vi "uActor_ReceiveNestedStopped.vi"(8 "error in (no error)":errorcluster, 10 "uData in":refnum<class "uData.lvclass">, 11 "uActor in":refnum<class "uActor.lvclass">) -> (0 "error out":errorcluster, 3 "uActor out":refnum<class "uActor.lvclass">)   [LabVIEW 2023, in "uLib.lvlib" / "uActor.lvclass"]
uses:
  uActor.lvclass
  uData/uData/uData.lvclass
  uData/uData/uData.lvclass/uData.ctl
  uActor.lvclass/uActor.ctl
  uData/uData/Condition Tag Name.vi
  uData/uData/Blank Key Reserved String.vi
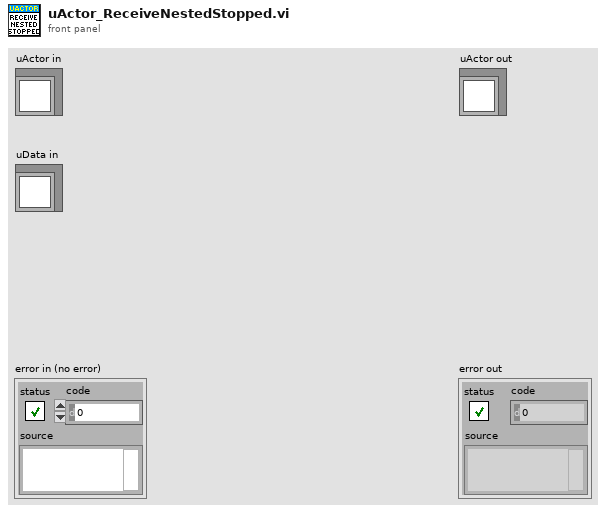
[diagram p1: front panel]
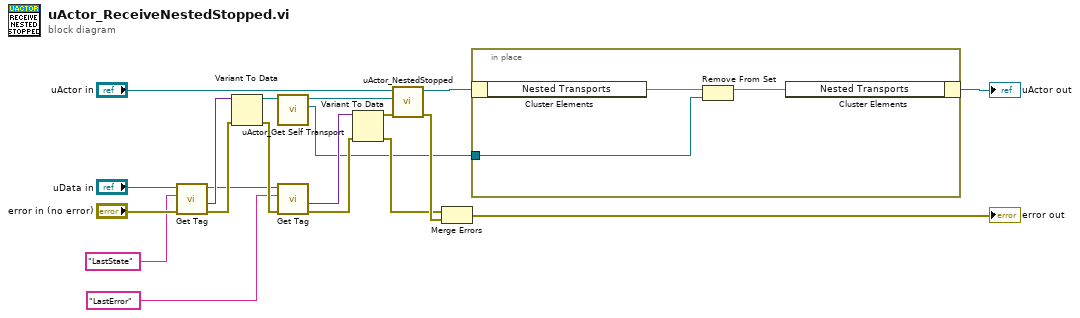
[diagram p0: block diagram]
diagram:
  n1 = call "Get Tag.vi"("error in (no error)"="error in (no error)", "tag (case insensitive)"="LastState" ("uMsg Tag"), "uData in"="uData in") -> ("error out"=w15:errorcluster, "value"=w18:variant, "uData out"=w13:refnum<class "uData.lvclass">)  [unwired: 5 in, 1 out]
  n2 = Variant To Data(error in=w15, Variant=w18) -> (data=w5:refnum<class "uActor.lvclass">, error out=w14:errorcluster)  [unwired: 1 in]
  n3 = call "uActor_Get Self Transport.vi"("uActor in"=w5) -> ("Actor Transport"=w3:refnum<class "uTransport_uActor.lvclass">, "uActor out"=w4:refnum<class "uActor.lvclass">)  [unwired: 9 in]
  n4 = call "Get Tag.vi"("error in (no error)"=w14, "tag (case insensitive)"="LastError" ("uMsg Tag"), "uData in"=w13) -> ("error out"=w12:errorcluster, "value"=w16:variant)  [unwired: 5 in, 2 out]
  n5 = Variant To Data(error in=w12, Variant=w16) -> (data=w17:errorcluster, error out=w11:errorcluster)  [unwired: 1 in]
  n6 = call-dynamic "uActor_NestedStopped.vi"("NestedActor - Last Error"=w17, "NestedActor - Last State"=w4, "uActor in"="uActor in") -> ("error out"=w19:errorcluster, "uActor out"=w7:refnum<class "uActor.lvclass">)  [unwired: 7 in]
  n7 = Merge Errors(w11, w19) -> (→"error out":errorcluster)
  n8 = in-place {
    in-place-border: w3 -> [w21]
    n9 = in-place-cluster #1(w7) -> ("Nested Transports"=w23:set{refnum<class "uTransport_uActor.lvclass">})
    n10 = Remove From Set(10:w21, 11:w23) -> (3:w22:set{refnum<class "uTransport_uActor.lvclass">})  [unwired: 1 out]
    n11 = in-place-cluster #1("Nested Transports"=w22) -> (→"uActor out":refnum<class "uActor.lvclass">)
  }
